vi "merge fault lists.vi"(10 "rt faults":T3[](array[typedef]), 11 "faults in":T1[](array[typedef])) -> (3 "faults out":T1[](array[typedef]))   [LabVIEW 2013, in "main engine.lvlib"]
uses:
  main engine/main engine.lvlib
  rt fault.ctl
  <vilib>/NI/Tag Bus Module Framework/runtime/error classification.ctl
  <vilib>/NI/Tag Bus Module Framework/module configuration/TBM module configuration.lvclass
  <vilib>/NI/Module Execution Interface/Engine Runtime/Fault.ctl
  <vilib>/NI/Configuration Framework/serializable configuration/NISE_CEF_serializable configuration.lvclass/NISE_CEF_serializable configuration.ctl
  <vilib>/NI/Configuration Framework/serializable configuration/NISE_CEF_serializable configuration.lvclass
  <vilib>/NI/Tag Bus Module Framework/runtime/TBM module execution interface.lvclass
  <vilib>/NI/Module Execution Interface/Engine Runtime/Engine Runtime Interface.lvclass
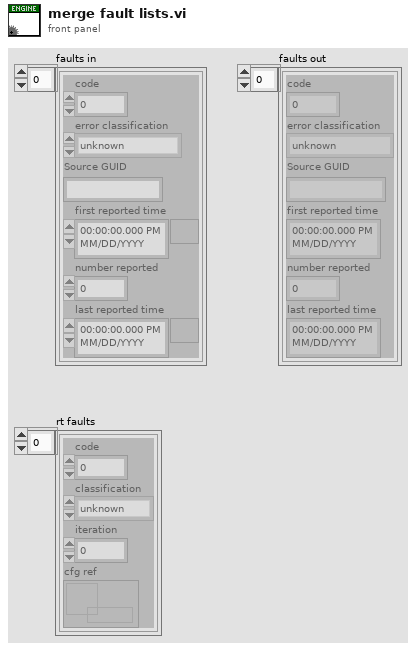
[diagram p1: front panel]
types:
  T1 = typedef "Engine Runtime Interface.lvclass/Fault.ctl" = cluster{"code":i32, "error classification":T2, "Source GUID":string, "first reported time":timestamp, "number reported":u32, "last reported time":timestamp}
  T2 = typedef "TBM module execution interface.lvclass/error classification.ctl" = enum16{"unknown", "none", "trivial", "recoverable", "critical"}
  T3 = typedef "main engine.lvlib/rt fault.ctl" = cluster{"code":i32, "classification":T2, "iteration":u64, "cfg ref":refnum<data-value>}
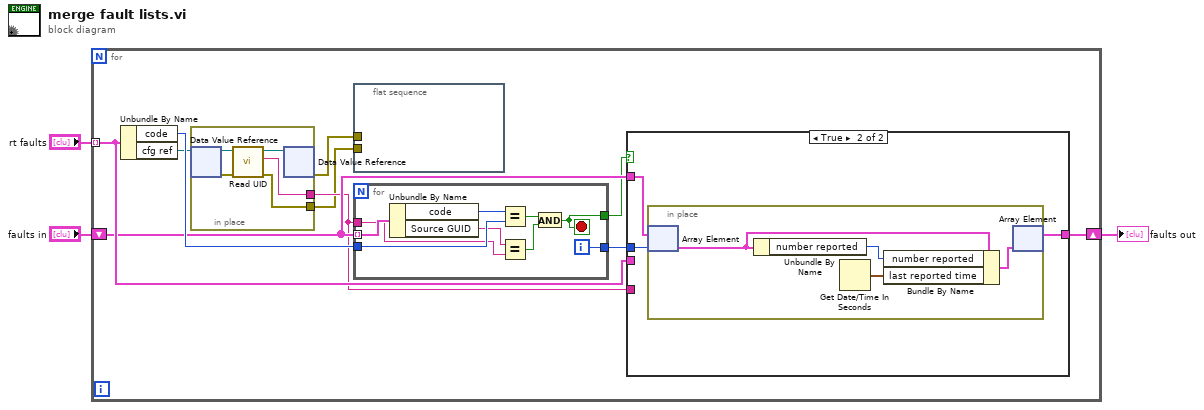
[diagram p0: block diagram]
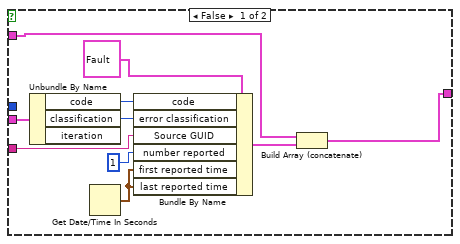
[diagram p2: hidden frame]
diagram:
  n1 = for {
    shift-right: [w10] -> w2
    shift-left: "faults in" -> [w11]
    tunnel: "rt faults" -> [w12] mode=indexing
    n2 = Unbundle By Name(w12) -> ("code"=w13:i32, "cfg ref"=w9:refnum<data-value>)
    n3 = in-place {
      in-place-border: [w41] -> w8
      in-place-border: [w40] -> w4
      n4 = in-place-dvr #1(w9) -> (w44:refnum<class "TBM module configuration.lvclass">, w42:errorcluster)
      n5 = call <vilib>:"Read UID.vi"("error in"=w42, "configuration in"=w44) -> ("error out"=w40:errorcluster, "instance id"=w41:string, "configuration out"=w43:refnum<class "TBM module configuration.lvclass">)  [unwired: 7 in]
      n6 = in-place-dvr #1(w43) -> (w5:errorcluster)  [unwired: 1 out]
    }
    n7 = flat-sequence {
      tunnel: w5 -> [_]
      tunnel: w4 -> [_]
      frame #0 {
      }
    }
    n8 = for {
      tunnel: w11 -> [w39] mode=indexing
      tunnel: w13 -> [w37]
      tunnel: w8 -> [w36]
      tunnel: [w32] -> w6
      tunnel: [w31] -> w7
      i -> [w32]
      stop <- w31 stop-if-true
      n9 = Unbundle By Name(w39) -> ("code"=w38:i32, "Source GUID"=w35:string)
      n10 = Equal?(x=w38, y=w37) -> (x = y?=w34:bool)
      n11 = Equal?(x=w35, y=w36) -> (x = y?=w33:bool)
      n12 = And(x=w34, y=w33) -> (x .and. y?=w31:bool)
    }
    n13 = case shown="True" w7 {
      tunnel: w12 -> [w19 _]
      tunnel: w8 -> [w16 _]
      tunnel: w6 -> [_ w25]
      tunnel: w11 -> [w23 w26]
      tunnel: [w22 w24] -> w10
      frame False {
        n14 = Unbundle By Name(w19) -> ("code"=w17:i32, "classification"=w18:T2)  [unwired: 1 out]
        n15 = Get Date/Time In Seconds() -> (seconds since 1Jan1904=w14:timestamp)
        n16 = Bundle By Name(cluster=T1 {"code"=0, "error classification"=enum."unknown", "Source GUID"="", "first reported time"=timestamp(0 s since 1904-01-01), "number reported"=0, "last reported time"=timestamp(0 s since 1904-01-01)} ("fault"), "code"=w17, "error classification"=w18, "Source GUID"=w16, "number reported"=u32 1, "first reported time"=w14, "last reported time"=w14) -> (w20:T1)
        n17 = Build Array (concatenate)(w23, w20) -> (w22:T1[])
      }
      frame True {
        n18 = in-place {
          n19 = in-place-array #2(w26, w25) -> (w30:T1)
          n20 = Unbundle By Name(w30) -> ("number reported"=w28:u32)
          n21 = Get Date/Time In Seconds() -> (seconds since 1Jan1904=w27:timestamp)
          n22 = Bundle By Name(cluster=w30, "number reported"=w28, "last reported time"=w27) -> (w29:T1)
          n23 = in-place-array #2(w29) -> (w24:T1[])  [unwired: 1 out]
        }
      }
    }
  }
  "faults out" <- w2
